vi "Read Config File.vi"(8 "error in (no error)":cluster{"状态":bool, "代码":i32, "源":string} caption="错误输入（无错误）", 11 "多任务通讯输入":refnum<class "多任务通讯.lvclass">) -> (0 "error out":cluster{"状态":bool, "代码":i32, "源":string} caption="错误输出", 3 "多任务通讯输出":refnum<class "多任务通讯.lvclass">)   [LabVIEW 2013, in "多任务通讯.lvlib" / "多任务通讯.lvclass"]
doc: "读取配置文件（如存在）内容，用于控制应用程序的运行。"
uses:
  <vilib>/Utility/config.llb/NI_LVConfig.lvlib
  <vilib>/Utility/config.llb/Read Key (I32).vi
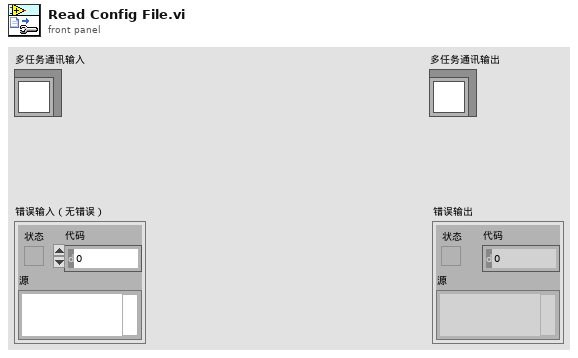
[diagram p1: front panel]
types:
  T1 = typedef "NI_LVConfig.lvlib/Config Data RefNum.ctl" = refnum<k1>
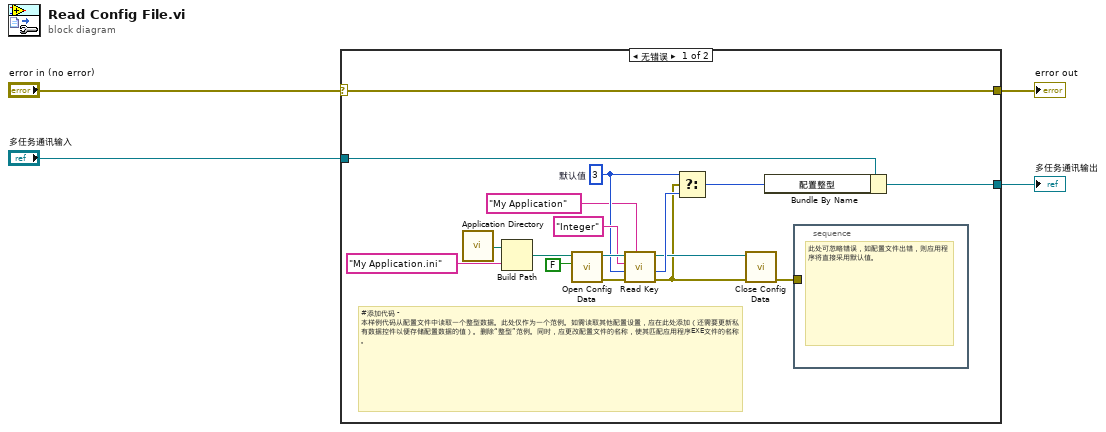
[diagram p0: block diagram]
diagram:
  n1 = case shown="无错误" "error in (no error)" {
    selector: "error in (no error)" -> [w6 w23]
    tunnel: [w6 w23] -> w3
    tunnel: [w10 w22] -> w1
    tunnel: "多任务通讯输入" -> [w11 w22]
    frame No Error {
      w14 = 3  # 默认值
      # "#添加代码 - 本样例代码从配置文件中读取一个整型数据。此处仅作为一个范例。如需读取其他配置设置，应在此处添加（还需要更新私有数据控件以便存储配置数据的值）。删除“整型”范例。同时，应更改配置文件的名称，使其匹配应用程序EXE文件的名称。"
      n2 = call <vilib>:"Application Directory.vi"() -> ("Application Directory"=w21:path)
      n3 = Build Path(base path=w21, name or relative path="My Application.ini") -> (appended path=w19:path)
      n4 = call <vilib>:"Open Config Data.vi"("create file if necessary (T)"=FALSE, "configuration file path"=w19) -> ("error out"=w17:errorcluster, "refnum"=w16:T1)  [unwired: 7 in, 1 out]
      n5 = call-poly <vilib>:"Read Key.vi"("section"="My Application", "error in (no error)"=w17, "default value"=w14, "key"="Integer", "refnum"=w16) -> ("error out"=w8:errorcluster, "value"=w13:i32, "refnum out"=w9:T1)  [unwired: 3 in, 1 out]
      n6 = Select(t=w14, s=w8, f=w13) -> (s? t:f=w12:i32)
      n7 = call <vilib>:"Close Config Data.vi"("error in (no error)"=w8, "refnum"=w9) -> ("error out"=w7:errorcluster)  [unwired: 8 in, 1 out]
      n8 = Bundle By Name(cluster=w11, "配置整型"=w12) -> (w10:refnum<class "多任务通讯.lvclass">)
      n9 = stacked-sequence {
        tunnel: w7 -> [_]
        frame #0 {
          # "此处可忽略错误，如配置文件出错，则应用程序将直接采用默认值。"
        }
      }
    }
    frame Error {
    }
  }
  "error out" <- w3
  "多任务通讯输出" <- w1
